vi "Eas_decryption.vi"(8 "Error In":errorcluster, 11 "Key":string) -> (0 "error out":errorcluster, 3 "Key":string)   [LabVIEW 2016]
uses:
  <vilib>/Alab Technologies/AES Crypto/Controls/Key Length.ctl
  <vilib>/Alab Technologies/AES Crypto/AES Crypto.lvlib
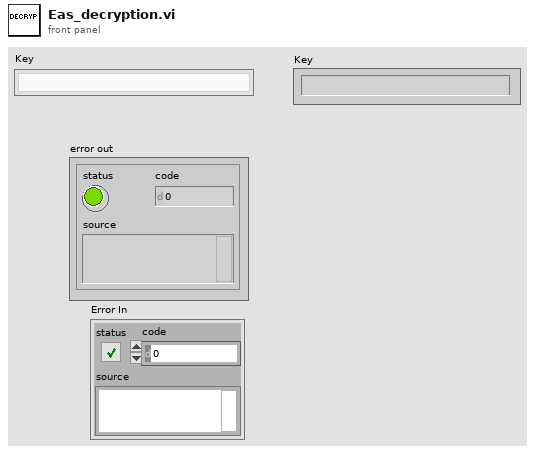
[diagram p1: front panel]
types:
  T1 = typedef "AES Crypto.lvlib/Key Length.ctl" = enum16{"128", "192", "256"}
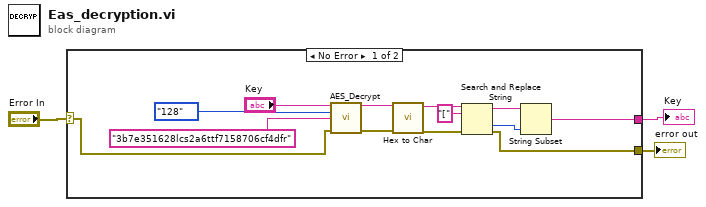
[diagram p0: block diagram]
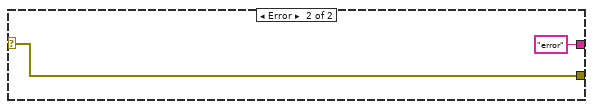
[diagram p2: hidden frame]
diagram:
  n1 = case shown="No Error" "Error In" {
    selector: "Error In" -> [w5 w17]
    tunnel: [w7 w17] -> w3
    tunnel: [w6 "error" ("result string")] -> w2
    frame No Error {
      n2 = call <vilib>:"AES_Decrypt.vi"("Cipher text (hex)"="Key", "Key length"=Key_Length."128", "Key (hex)"="3b7e351628lcs2a6ttf7158706cf4dfr", "Error In"=w5) -> ("Plain text (hex)"=w15:string, "Error out"=w16:errorcluster)  [unwired: 10 in]
      n3 = call <vilib>:"Hex to Char.vi"("Input string (hex)"=w15, "error in (no error)"=w16) -> ("Output string (char)"=w11:string, "error out"=w8:errorcluster)  [unwired: 12 in]
      n4 = Search and Replace String(input string=w11, search string="[", error in=w8) -> (result string=w9:string, offset past replacement=w4:i32, error out=w7:errorcluster)  [unwired: 5 in, 1 out]
      n5 = String Subset(string=w9, length (rest)=w4) -> (substring=w6:string)  [unwired: 1 in]
    }
    frame Error {
    }
  }
  "error out" <- w3
  "Key" <- w2
